vi "releasePresure.vi"(9 "targetPressure":dbl, 10 "maximumTolerance":dbl, 11 "minimumTolerance":dbl) -> (2 "current pr":dbl, 3 "maximumPressure":dbl format="%0.2f")   [LabVIEW 2015]
uses:
  EFCO VIs/Control test 1.ctl
  <vilib>/wsapi/Web Request.lvclass
  <vilib>/Waveform/WDTOps.llb/WDT Append Waveforms DBL.vi
panel:
  in  "LabVIEW Web Service Request":refnum<class "Web Request.lvclass">
  out "value":string
  in  "stop (F)":bool
  out "data":T1
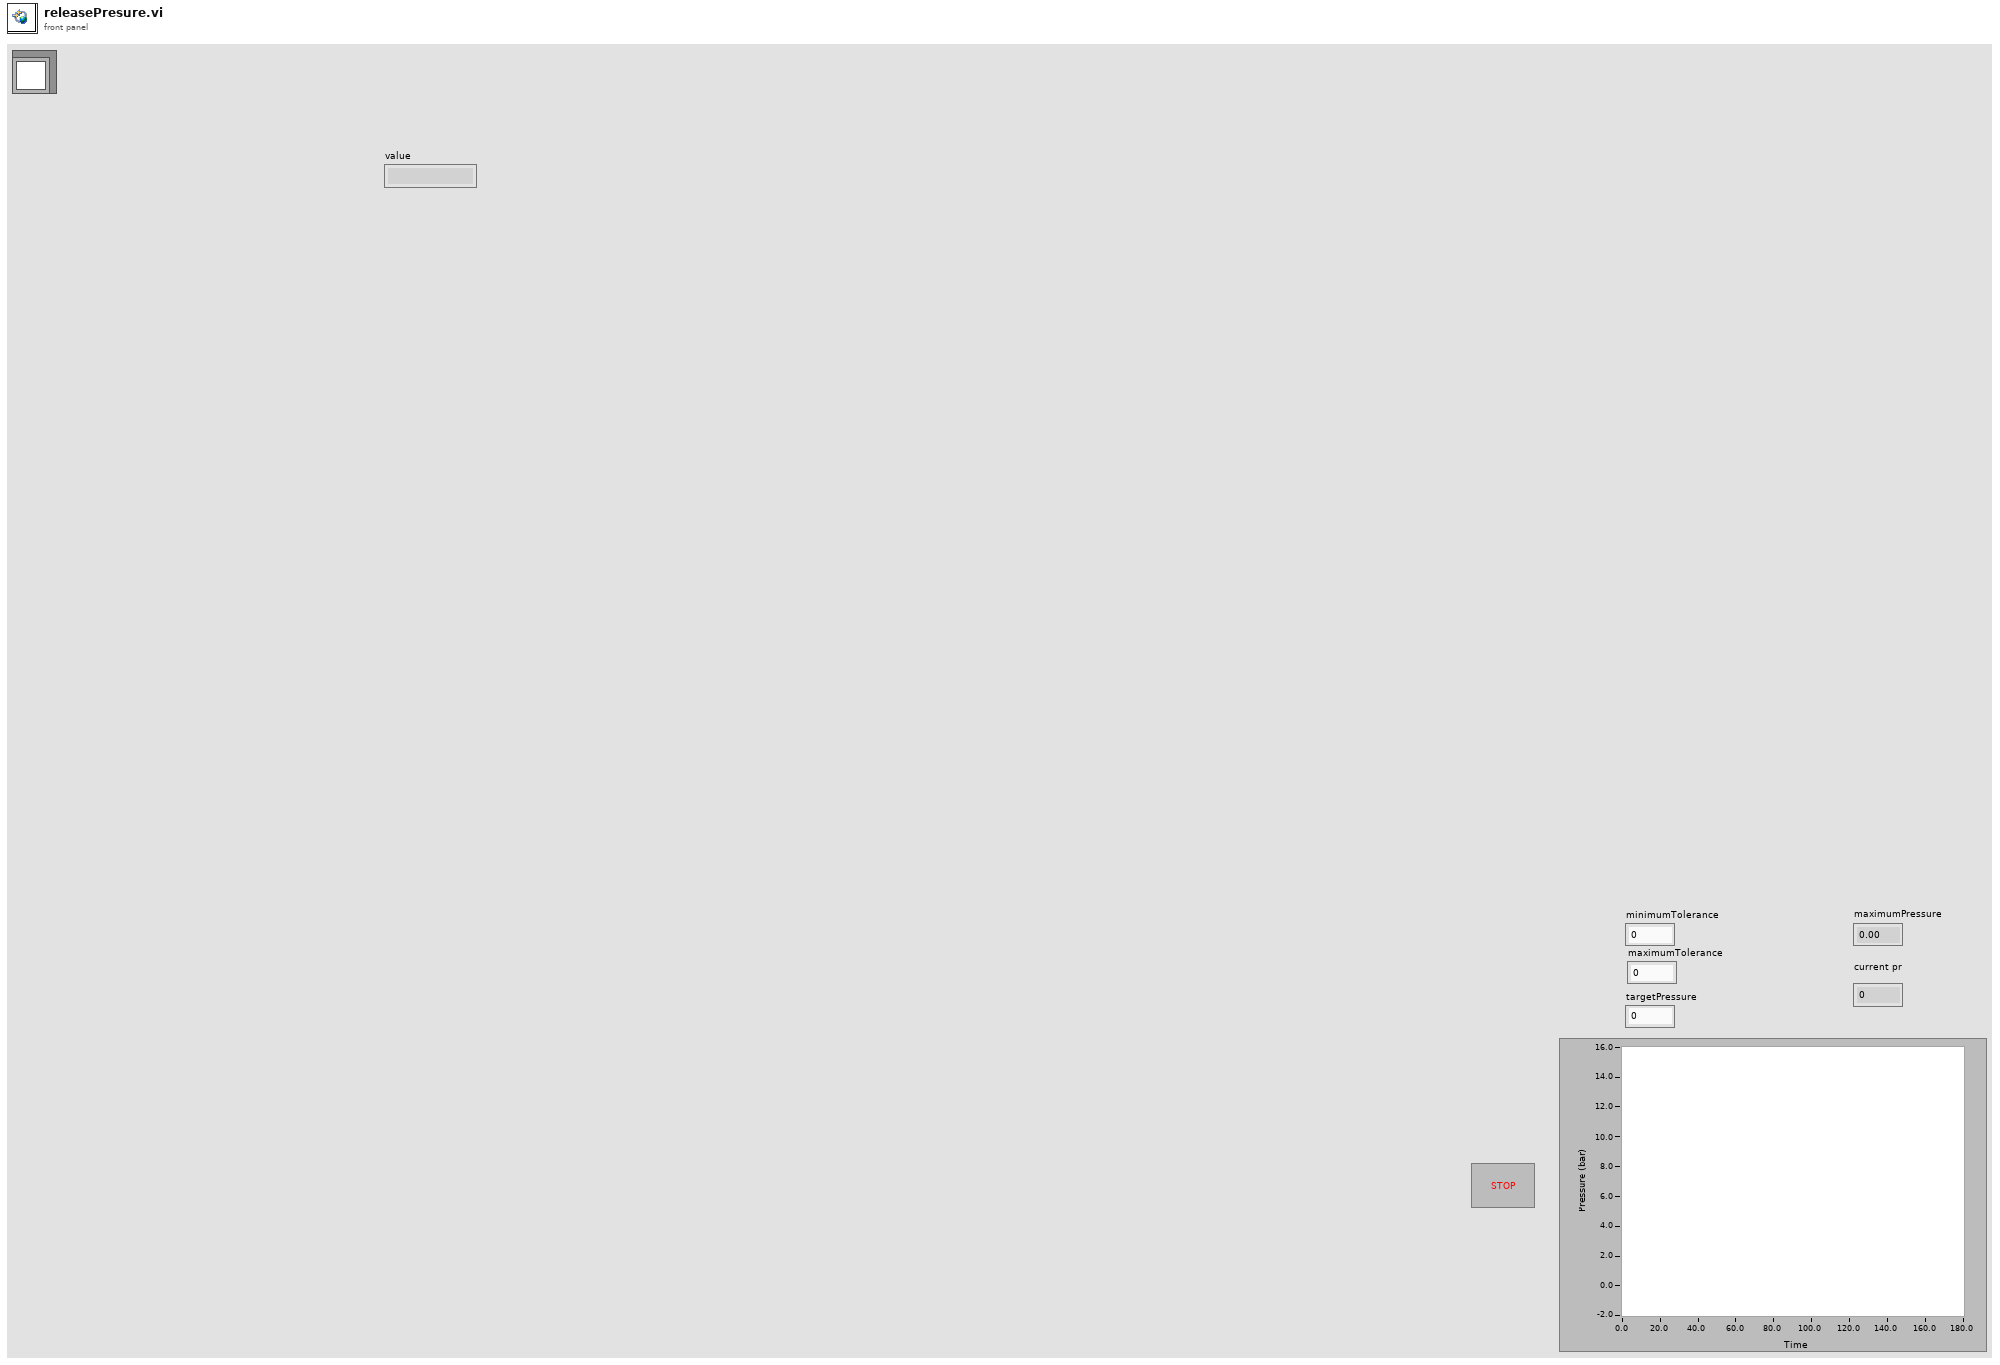
[diagram p1: front panel]
types:
  T1 = typedef "Control test 1.ctl" = dynamicdata
  T2 = typedef "imagedata.ctl" = cluster{"image type":i32, "image depth":i32, "image":u8[], "mask":u8[], "colors":u32[], "Rectangle":cluster{"left":i16, "top":i16, "right":i16, "bottom":i16}}
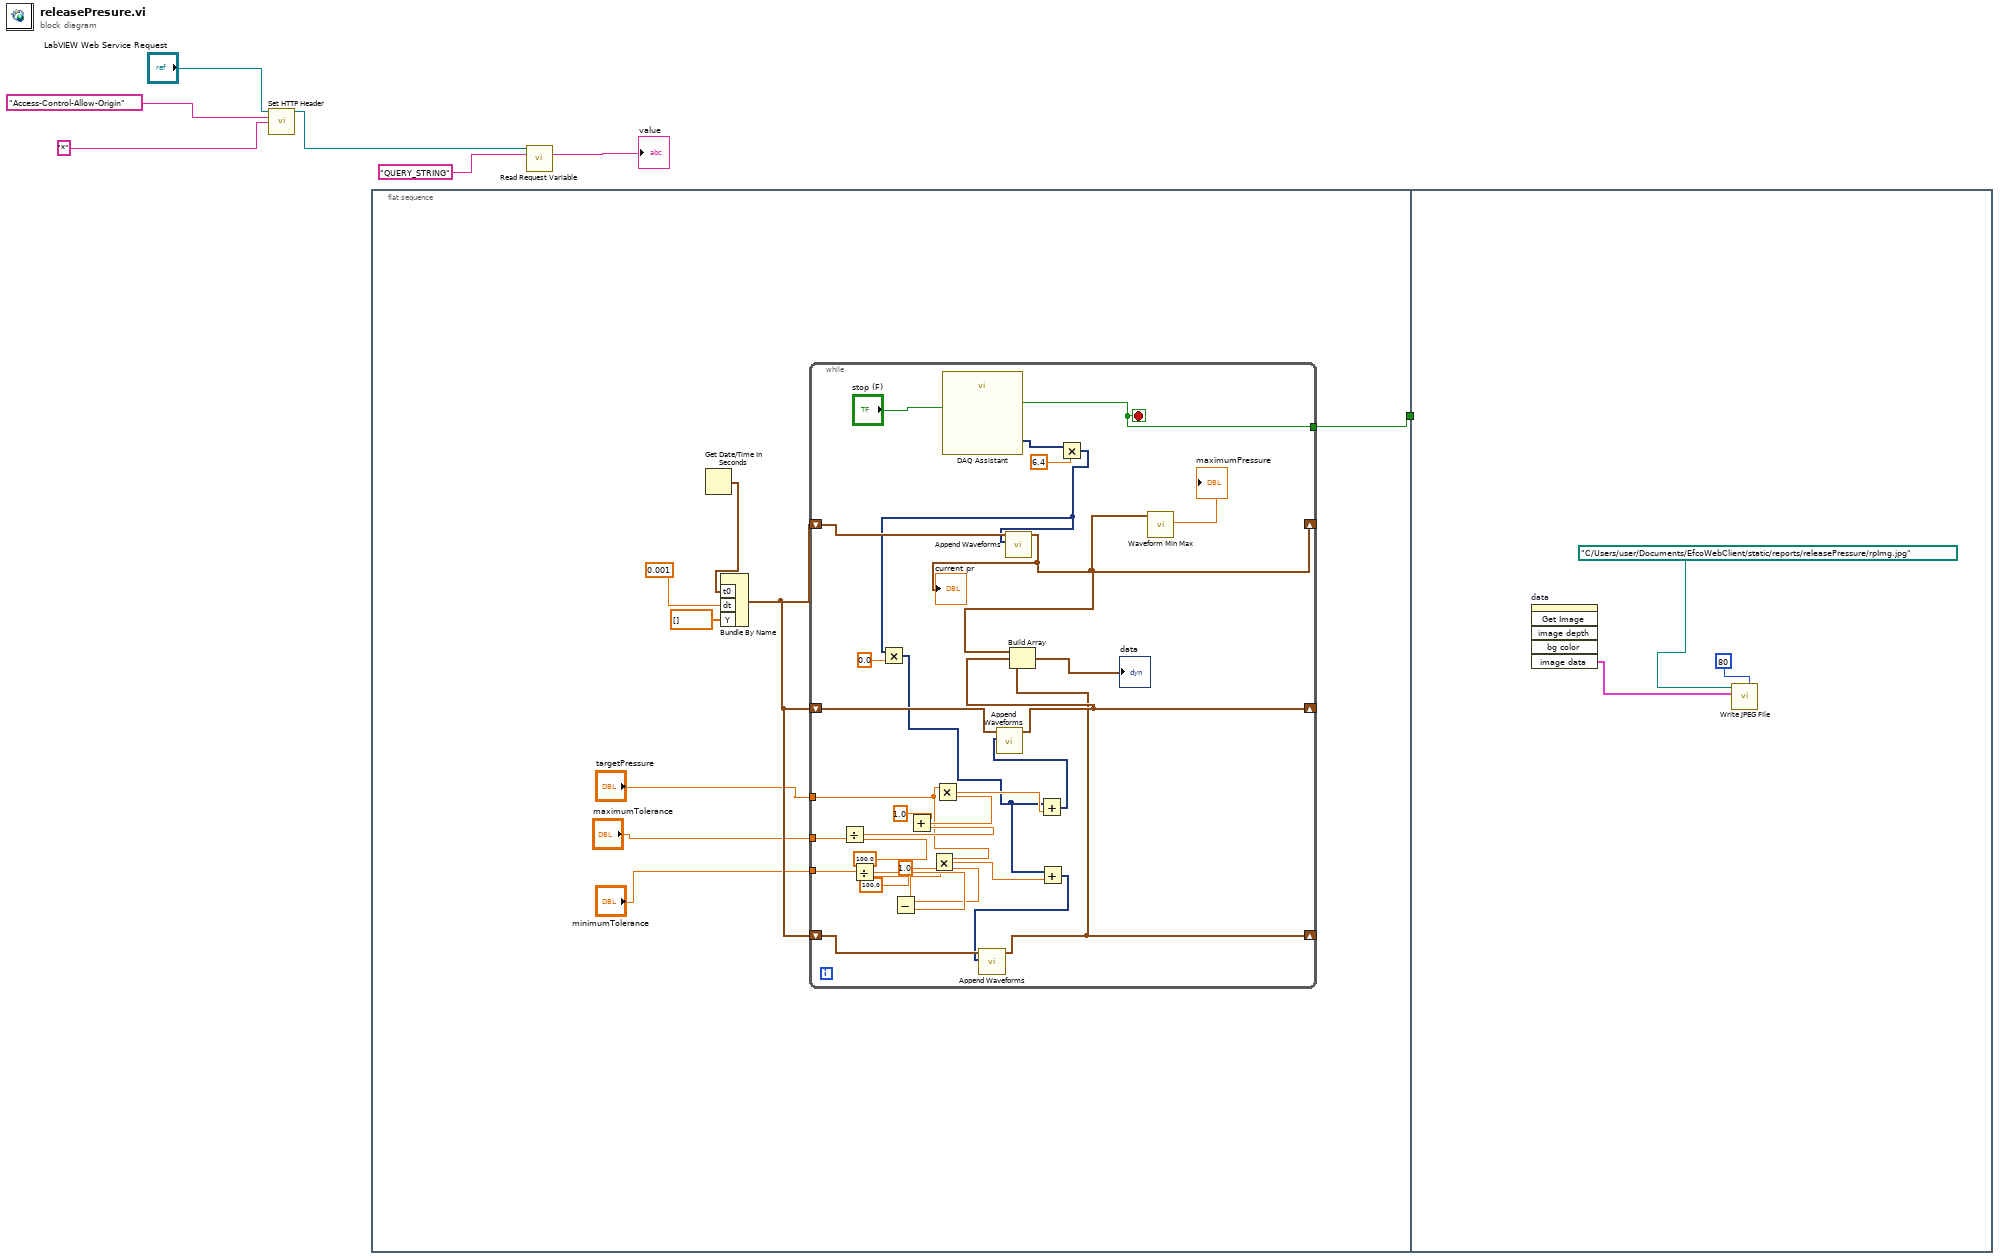
[diagram p0: block diagram]
diagram:
  n1 = call <vilib>:"Set HTTP Header.vi"("LabVIEW Web Service Request"="LabVIEW Web Service Request", "header"="Access-Control-Allow-Origin", "header value"="*") -> ("LabVIEW Web Service Request out"=w2:refnum<class "Web Request.lvclass">)  [unwired: 11 in, 1 out]
  n2 = flat-sequence {
    tunnel: [w8] -> w7
    tunnel: w7 -> [_]
    frame #0 {
      n3 = Get Date/Time In Seconds() -> (seconds since 1Jan1904=w14:timestamp)
      n4 = Bundle By Name("t0"=w14, "dt"=0.001, "Y"=dbl[] []) -> (w13:waveform(dbl))  [unwired: 1 in]
      n5 = while {
        shift-right: [w19] -> _
        shift-left: w13 -> [w22]
        shift-right: [w42] -> _
        shift-left: w13 -> [w43]
        tunnel: "maximumTolerance" -> [w41]
        tunnel: "minimumTolerance" -> [w39]
        tunnel: "targetPressure" -> [w31]
        shift-right: [w18] -> _
        shift-left: w13 -> [w27]
        tunnel: [w16] -> w8
        stop <- w16 stop-if-true
        n6 = Divide(x=w41, y=100.0) -> (x/y=w36:dbl)
        n7 = Divide(x=w39, y=100.0) -> (x/y=w35:dbl)
        n8 = Subtract(x=1.0, y=w35) -> (x-y=w33:dbl)
        n9 = Add(x=1.0, y=w36) -> (x+y=w32:dbl)
        n10 = Multiply(x=w31, y=w33) -> (x*y=w25:dbl)
        n11 = Multiply(x=w31, y=w32) -> (x*y=w29:dbl)
        n12 = call "DAQ Assistant"("stop (F)"="stop (F)") -> ("data"=w23:dynamicdata, "stopped"=w16:bool)  [unwired: 15 in, 2 out]
        n13 = Multiply(x=w23, y=6.4) -> (x*y=w20:dynamicdata)
        n14 = Multiply(x=w20, y=0.0) -> (x*y=w26:dynamicdata)
        n15 = call-poly <vilib>:"Append Waveforms.vi"("waveform B"=w20, "waveform A"=w22) -> ("waveform out"=w19:waveform(dbl))  [unwired: 8 in, 1 out]
        "current pr" <- w19
        n16 = Add(x=w26, y=w29) -> (x+y=w28:dynamicdata)
        n17 = call-poly <vilib>:"Append Waveforms.vi"("waveform B"=w28, "waveform A"=w43) -> ("waveform out"=w42:waveform(dbl))  [unwired: 8 in, 1 out]
        n18 = Add(x=w26, y=w25) -> (x+y=w24:dynamicdata)
        n19 = call-poly <vilib>:"Append Waveforms.vi"("waveform B"=w24, "waveform A"=w27) -> ("waveform out"=w18:waveform(dbl))  [unwired: 8 in, 1 out]
        n20 = Build Array(w19, w42, w18) -> (→"data":waveform(dbl)[])
        n21 = call <vilib>:"Waveform Min Max.vi"("waveform in"=w19) -> ("Y max"=→"maximumPressure":dbl)  [unwired: 5 in, 5 out]
      }
    }
    frame #1 {
      n22 = invoke on="data" class="WFGraph (strict)" method="Get Image"() -> ("image data"=w48:T2)  [unwired: 6 in, 5 out]
      n23 = call <vilib>:"Write JPEG File.vi"("quality (80)"=80, "image data"=w48, "path to JPEG file"=path "C:/Users/user/Documents/EfcoWebClient/static/reports/releasePressure/rpImg.jpg") -> ()  [unwired: 7 in, 2 out]
    }
  }
  n24 = call <vilib>:"Read Request Variable.vi"("LabVIEW Web Service Request"=w2, "variable name"="QUERY_STRING") -> ("value"=→"value":string)  [unwired: 11 in, 2 out]
